vi "InitializeLine.vi"(2 "Store Data":bool, 3 "Image Settings":T1={"Start Position (µm)"={"x"=0.0, "y"=0.0, "z"=0.0}, "End Position (µm)"={"x"=10.0, "y"=10.0, "z"=0.0}, "Image Resolution (nm/pixel)"={"x"=50.0, "y"=50.0, "z"=100.0}, "Image Size (µm)"={"x"=10.0, "y"=10.0, "z"=0.0}, "Image Size (pixel)"={"x"=50, "y"=50, "z"=0}, "Time Resolution\n(ms/pixel)"=7.0, "1st Axis"=0, "2nd Axis"=1, "Retrace"=FALSE, "Estimated Time"=""} {"2nd Axis" items=["x", "y", "z"]; "1st Axis" items=["x", "y", "z"]; "Time Resolution\n(ms/pixel)" format="%.2f"; "Image Resolution (nm/pixel)"."z" format="%.2f"; "Image Resolution (nm/pixel)"."y" format="%.2f"; "Image Resolution (nm/pixel)"."x" format="%.2f"; "Image Size (µm)"."z" format="%.2f"; "Image Size (µm)"."y" format="%.2f"; "Image Size (µm)"."x" format="%.2f"; "End Position (µm)"."z" format="%.2f"; "End Position (µm)"."y" format="%.2f"; "End Position (µm)"."x" format="%.2f"; "Start Position (µm)"."z" format="%.2f"; "Start Position (µm)"."y" format="%.2f"; "Start Position (µm)"."x" format="%.2f"}, 4 "error in (no error)":errorcluster, 5 "Destination:":path) -> (0 "error out":errorcluster, 1 "Busy":bool)   [LabVIEW 2009]
uses:
  ImageSettings.ctt
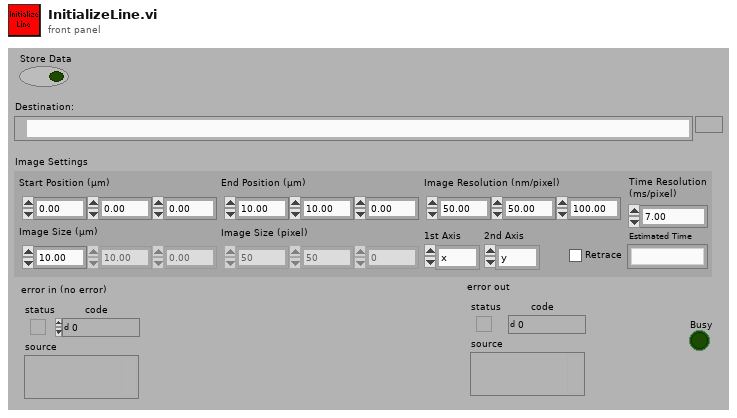
[diagram p1: front panel]
types:
  T1 = typedef "ImageSettings.ctt" = cluster{"Start Position (µm)":cluster{"x":dbl, "y":dbl, "z":dbl}, "End Position (µm)":cluster{"x":dbl, "y":dbl, "z":dbl}, "Image Resolution (nm/pixel)":cluster{"x":dbl, "y":dbl, "z":dbl}, "Image Size (µm)":cluster{"x":dbl, "y":dbl, "z":dbl}, "Image Size (pixel)":cluster{"x":u32, "y":u32, "z":u32}, "Time Resolution\n(ms/pixel)":dbl, "1st Axis":u16, "2nd Axis":u16, "Retrace":bool, "Estimated Time":string}
  T2 = typedef "LineScanStatus.ctt" = cluster{"in line":bool, "line status":cluster{"count":u32, "current":cluster{"x":u32, "y":u32, "z":u32}}, "plane status":cluster{"count":u32, "current":cluster{"x":u32, "y":u32, "z":u32}}, "new line step":cluster{"x":dbl, "y":dbl, "z":dbl}, "new plane step":cluster{"x":dbl, "y":dbl, "z":dbl}}
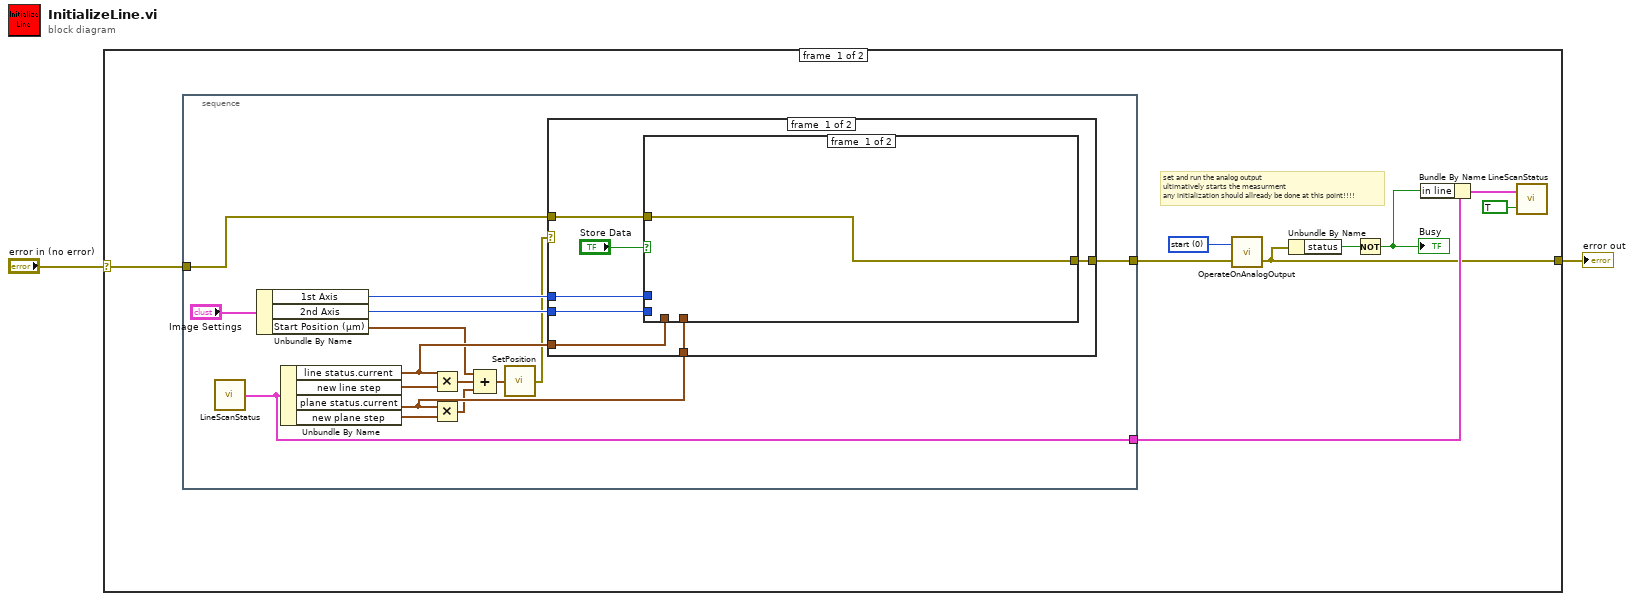
[diagram p0: block diagram]
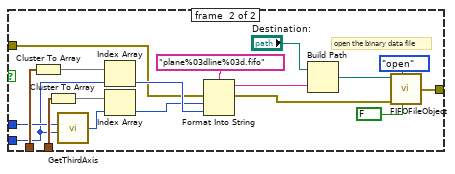
[diagram p2: hidden frame]
diagram:
  n1 = case shown="No Error" "error in (no error)" {
    selector: "error in (no error)" -> [w6 w54]
    tunnel: [w7 w54] -> w2
    frame #0 {
      w5 = u16 0 items=["start", "state", "abort"] ("operation")
      # "set and run the analog output\nultimatively starts the measurment\nany initialization should allready be done at this point!!!!"
      n2 = stacked-sequence {
        tunnel: [w21] -> w9
        tunnel: w6 -> [w20]
        tunnel: [w13] -> w3
        frame #0 {
          n3 = call "LineScanStatus.vi"() -> ("Linescan Status (output)"=w21:T2)  [unwired: 2 in]
          n4 = Unbundle By Name("Image Settings") -> ("1st Axis"=w19:u16, "2nd Axis"=w18:u16, "Start Position (µm)"=w17:cluster{"x":dbl, "y":dbl, "z":dbl})
          n5 = Unbundle By Name(w21) -> ("line status.current"=w23:cluster{"x":u32, "y":u32, "z":u32}, "new line step"=w25:cluster{"x":dbl, "y":dbl, "z":dbl}, "plane status.current"=w22:cluster{"x":u32, "y":u32, "z":u32}, "new plane step"=w24:cluster{"x":dbl, "y":dbl, "z":dbl})
          n6 = Multiply(x=w23, y=w25) -> (x*y=w16:cluster{"x":dbl, "y":dbl, "z":dbl})
          n7 = Multiply(x=w22, y=w24) -> (x*y=w15:cluster{"x":dbl, "y":dbl, "z":dbl})
          n8 = Compound Arithmetic op=ADD(w17, w16, w15) -> (w14:cluster{"x":dbl, "y":dbl, "z":dbl})
          n9 = call "SetPosition.vi"("Current Position (µm)"=w14) -> ("error out"=w12:errorcluster)
          n10 = case shown="No Error" w12 {
            selector: w12 -> [_ w53]
            tunnel: w23 -> [w33 _]
            tunnel: w22 -> [w32 _]
            tunnel: w20 -> [w31 _]
            tunnel: w19 -> [w30 _]
            tunnel: w18 -> [w29 _]
            tunnel: [w28 w53] -> w13
            frame #0 {
              n11 = case shown="True" "Store Data" {
                tunnel: w33 -> [_ w52]
                tunnel: w32 -> [_ w51]
                tunnel: w31 -> [w34 w45]
                tunnel: w30 -> [_ w44]
                tunnel: w29 -> [_ w43]
                tunnel: [w34 w36] -> w28
                frame #0 {
                }
                frame #1 {
                  # "open the binary data file"
                  n12 = Cluster To Array(cluster=w52) -> (array=w48:u32[])
                  n13 = Cluster To Array(cluster=w51) -> (array=w47:u32[])
                  n14 = call "GetThirdAxis.vi"("1st Axis"=w43, "2nd Axis"=w44) -> ("3rd Axis"=w46:i32)  [unwired: 2 in]
                  n15 = Index Array(array=w48, index=w43) -> (element=w50:u32)
                  n16 = Index Array(array=w47, index=w46) -> (element=w49:u32)
                  n17 = Format Into String(format string="plane%03dline%03d.fifo", error in=w45, w49, w50) -> (resulting string=w41:string, error out=w37:errorcluster)  [unwired: 1 in]
                  n18 = Build Path(base path="Destination:", name or relative path=w41) -> (appended path=w42:path)
                  n19 = call "FIFOFileObject.vi"(".sm file format"=FALSE, "function (open:0)"=enum16{"open", "write", "close"}."open", "error in (no error)"=w37, "Destination:"=w42) -> ("error out"=w36:errorcluster)  [unwired: 2 in]
                }
              }
            }
            frame #1 {
            }
          }
        }
      }
      n20 = call "OperateOnAnalogOutput.vi"("error in (no error)"=w3, "operation"=w5) -> ("error out"=w7:errorcluster)  [unwired: 1 out]
      n21 = Unbundle By Name(w7) -> ("status"=w4:bool)
      n22 = Not(x=w4) -> (.not. x?=w8:bool)
      "Busy" <- w8
      n23 = Bundle By Name(cluster=w9, "in line"=w8) -> (w10:T2)
      n24 = call "LineScanStatus.vi"("Get/Set"=TRUE, "Linescan Status (input)"=w10) -> ()  [unwired: 1 out]
    }
    frame #1 {
    }
  }
  "error out" <- w2
